vi "Close VI.vi"(10 "VI Refnum":refnum<vi>, 11 "App Ref":refnum<vi>) -> ()   [LabVIEW 2024, in "Word Search Scorer.lvlib"]
uses:
  Word Search Scorer.lvlib
panel:
  out "tskill output":string
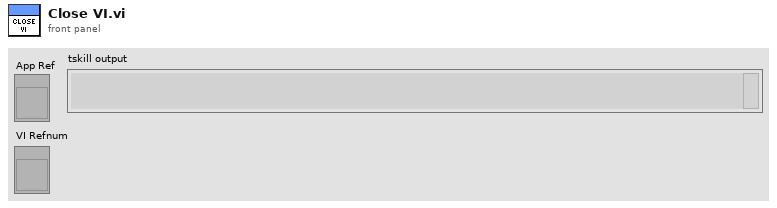
[diagram p1: front panel]
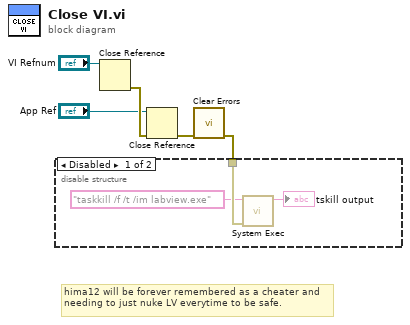
[diagram p0: block diagram]
diagram:
  # "hima12 will be forever remembered as a cheater and needing to just nuke LV everytime to be safe."
  n1 = Close Reference(reference="VI Refnum") -> (error out=w4:errorcluster)  [unwired: 1 in]
  n2 = Close Reference(reference="App Ref", error in (no error)=w4) -> (error out=w1:errorcluster)
  n3 = call <vilib>:"Clear Errors.vi"("error in (no error)"=w1) -> ("error out"=w5:errorcluster)  [unwired: 5 in, 1 out]
  n4 = disable-structure shown="Disabled" {
    disable-tunnel: w5 -> [w8 _]
    frame Disabled {
      n5 = call <vilib>:"System Exec.vi"("error in (no error)"=w8, "command line"="taskkill /f /t /im labview.exe") -> ("standard output"=→"tskill output":string)  [unwired: 6 in, 3 out]
    }
    frame Enabled {
    }
  }
